vi "Update Check-out Details.vi"(0 "Guest Manager UI in":refnum<class "Guest Manager UI.lvclass">, 5 "Guest Contact Number":string, 7 "Primary Guest Name":string, 9 "Bill Summary":string, 11 "error in (no error)":errorcluster) -> (4 "Guest Manager UI out":refnum<class "Guest Manager UI.lvclass">, 15 "error out":errorcluster)   [LabVIEW 2023, in "Guest Manager UI.lvlib" / "Guest Manager UI.lvclass"]
uses:
  Guest Manager UI.lvclass
  Guest Manager UI.lvclass/Guest Manager UI.ctl
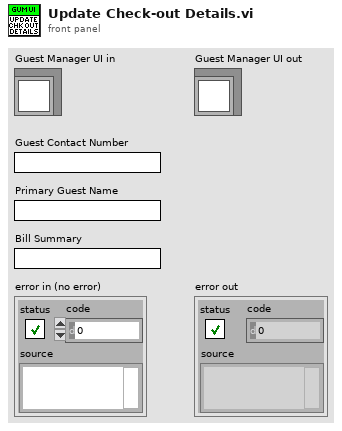
[diagram p1: front panel]
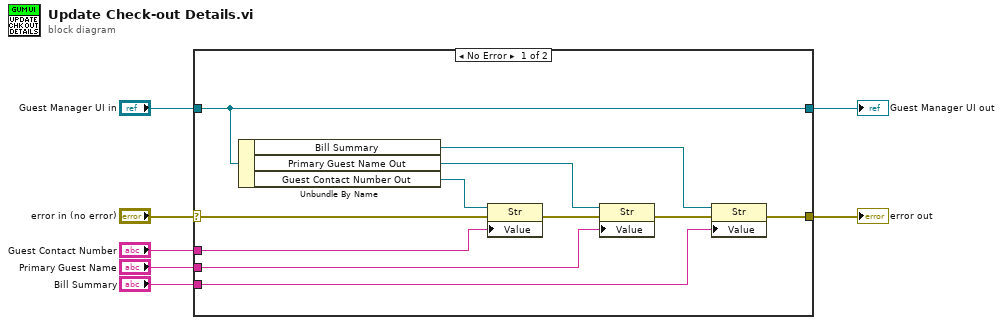
[diagram p0: block diagram]
diagram:
  n1 = case shown="No Error" "error in (no error)" {
    selector: "error in (no error)" -> [w18 w20]
    tunnel: [w12 w20] -> w6
    tunnel: [w17 w19] -> w4
    tunnel: "Guest Manager UI in" -> [w17 w19]
    tunnel: "Guest Contact Number" -> [w15 _]
    tunnel: "Primary Guest Name" -> [w9 _]
    tunnel: "Bill Summary" -> [w8 _]
    frame No Error {
      n2 = Unbundle By Name(w17) -> ("Bill Summary"=w10:refnum<vi>, "Primary Guest Name Out"=w11:refnum<vi>, "Guest Contact Number Out"=w16:refnum<vi>)
      n3 = property class="Str"(reference=w16, error in=w18, "Value"=w15) -> (error out=w14:errorcluster)  [unwired: 1 out]
      n4 = property class="Str"(reference=w11, error in=w14, "Value"=w9) -> (error out=w13:errorcluster)  [unwired: 1 out]
      n5 = property class="Str"(reference=w10, error in=w13, "Value"=w8) -> (error out=w12:errorcluster)  [unwired: 1 out]
    }
    frame Error {
    }
  }
  "error out" <- w6
  "Guest Manager UI out" <- w4
